vi "M09 Hydro pool - Copy.vi"(11 "EV3 in":T1) -> (3 "NXT/EV3":T1)   [LabVIEW 2016]
uses:
  <vilib>/NXT/Subs/LVHSConnector.ctl
  <vilib>/NXT/LegoClasses/BrickReference/BrickReference.lvclass
  <vilib>/NXT/Dual Mode Library/Waits/Wait_Num.vi
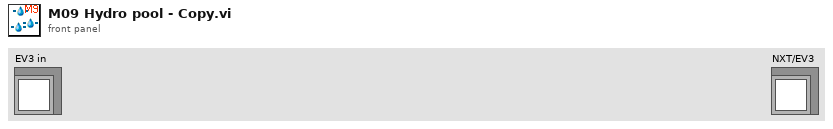
[diagram p1: front panel]
types:
  T1 = typedef "LVHSConnector.ctl" = refnum<class "BrickReference.lvclass">
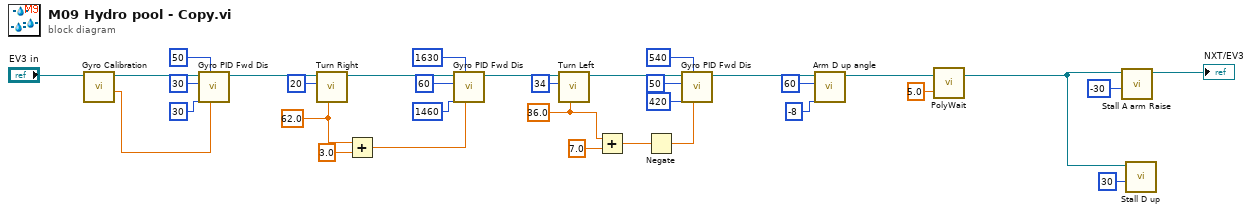
[diagram p0: block diagram]
diagram:
  w7 = sgl 36.0 ("Turning angle")
  w19 = sgl 62.0 ("Turning angle")
  n1 = call "Gyro Calibration.vi"("NXT/EV3"="EV3 in") -> ("Degrees"=w20:sgl, "NXT/EV3"=w21:T1)  [unwired: 6 in, 1 out]
  n2 = call "Gyro PID Fwd Dis.vi"("Target angle"=w20, "Threshold to stop"=50, "Threshold to slow"=30, "Max. speed"=30, "EV3 in"=w21) -> ("EV3 out"=w30:T1)  [unwired: 6 in]
  n3 = call "Turn Right.vi"("Turning angle"=w19, "Motor B (right)"=i8 20, "EV3 in"=w30) -> ("EV3 out"=w25:T1)  [unwired: 8 in]
  n4 = Add(x=w19, y=sgl 3.0) -> (x+y=w12:sgl)
  n5 = call "Gyro PID Fwd Dis.vi"("Target angle"=w12, "Threshold to stop"=1630, "Threshold to slow"=1460, "Max. speed"=60, "EV3 in"=w25) -> ("EV3 out"=w11:T1)  [unwired: 6 in]
  n6 = call "Turn Left.vi"("Turning angle"=w7, "Motor B (right)"=i8 34, "EV3 in"=w11) -> ("EV3 out"=w9:T1)  [unwired: 8 in]
  n7 = Add(x=w7, y=sgl 7.0) -> (x+y=w6:sgl)
  n8 = Negate(x=w6) -> (-x=w5:sgl)
  n9 = call "Gyro PID Fwd Dis.vi"("Target angle"=w5, "Threshold to stop"=540, "Threshold to slow"=420, "Max. speed"=50, "EV3 in"=w9) -> ("EV3 out"=w3:T1)  [unwired: 6 in]
  n10 = call "Arm D up angle.vi"("Power"=i8 -8, "Rotation"=60, "EV3 in"=w3) -> ("EV3 out"=w4:T1)  [unwired: 8 in]
  n11 = call-poly <vilib>:"PolyWait.vi"("Time (1 sec)"=sgl 5.0, "NXT/EV3"=w4) -> ("NXT/EV3"=w2:T1)  [unwired: 2 in]
  n12 = call "Stall A arm Raise.vi"("Power"=i8 -30, "NXT/EV3"=w2) -> ("NXT/EV3"=→"NXT/EV3":T1)  [unwired: 9 in]
  n13 = call "Stall D up.vi"("Power"=i8 30, "NXT/EV3"=w2) -> ()  [unwired: 9 in, 1 out]
